vi "i q sum.vi"(9 "input valid":bool=TRUE, 10 "data in":T1, 11 "data in":T1) -> (2 "output valid":bool, 3 "output cluster":T1)   [LabVIEW 2021]
doc: "sum 2 IQ datas (I+I =>I ; Q+Q =>Q ; overflow or overflow or +overflow => overflow"
uses:
  <instrlib>/_niInstr/DSP/v1/Shared/Public/IQ Data.ctl
  <vilib>/rvi/FXPMathLib/FxpAdd/XNode/nifxpmath_Add.xnode
  <vilib>/rvi/FXPMathLib/sim/FxpSim.dll
  <instrlib>/_niInstr/DSP/v1/Shared/niInstr DSP v1 Shared.lvlib
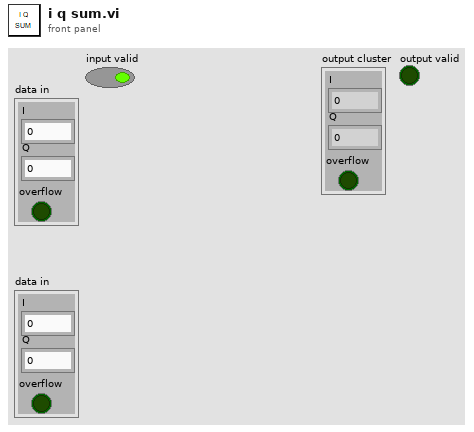
[diagram p1: front panel]
types:
  T1 = typedef "niInstr DSP v1 Shared.lvlib/IQ Data.ctl" = cluster{"I":fxp<+/-,18,1>, "Q":fxp<+/-,18,1>, "overflow":bool}
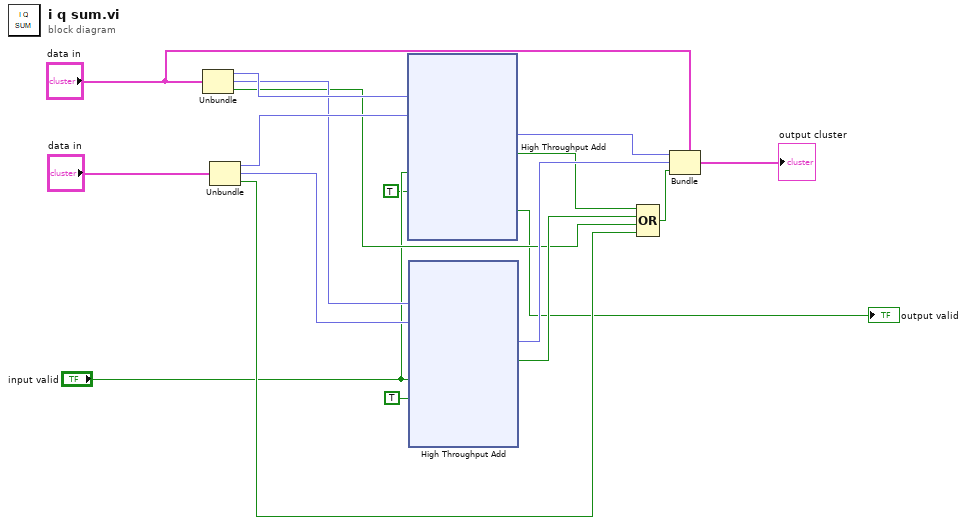
[diagram p0: block diagram]
diagram:
  n1 = Unbundle("data in") -> ("I"=w17:fxp<+/-,18,1>, "Q"=w15:fxp<+/-,18,1>, "overflow"=w9:bool)
  n2 = Unbundle("data in") -> ("I"=w16:fxp<+/-,18,1>, "Q"=w14:fxp<+/-,18,1>, "overflow"=w8:bool)
  n3 = xnode ("High Throughput Add")("x"=w17, "y"=w16, "input valid"="input valid", "ready for output (T)"=TRUE) -> ("x+y"=w13:fxp<+/-,18,1>, "operation overflow"=w11:bool, "output valid"=→"output valid":bool)  [unwired: 1 out]
  n4 = xnode ("High Throughput Add")("x"=w15, "y"=w14, "input valid"="input valid", "ready for output (T)"=TRUE) -> ("x+y"=w12:fxp<+/-,18,1>, "operation overflow"=w10:bool)  [unwired: 2 out]
  n5 = Compound Arithmetic op=OR(w11, w10, w9, w8) -> (w7:bool)
  n6 = Bundle(cluster="data in", "I"=w13, "Q"=w12, "overflow"=w7) -> (→"output cluster":T1)
